vi "Read ADU Packet Slave.vi"(7 "Slave (F)":bool, 8 "error in (no error)":errorcluster, 10 "Transaction ID WR":u16, 11 "TCP in":refnum<class "TCP.lvclass">) -> (0 "error out":errorcluster, 1 "Modbus Data Unit":T2={"function"=1, "Data"=[]} {"function" items=["Read Discrete Inputs"=2, "Read Coils"=1, "Write Single Coil"=5, "Write Multiple Coils"=15, "Read Input Register"=4, "Read Holding Registers"=3, "Write Single Register"=6, "Write Multiple Registers"=16, "Read/Write Multiple Registers"=23, "Mask Write Register"=22, "Read FIFO Queue"=24, "Read File Record"=20, "Write File Record"=21, "Read Exception Status"=7, "Diagnostic"=8, "Get Com Event Counter"=11, "Get Com Event Log"=12, "Report Slave ID"=17, "Read Device Identification"=43]; "Data" format="%.0x"}, 2 "MBAP Header":T1, 3 "TCP out":refnum<class "TCP.lvclass">, 5 "PDU Valid?":bool)   [LabVIEW 2019]
doc: "This uses the protocol layer to read a modbus packet off of the bus, wrapped in the IP transmission data unit."
uses:
  <vilib>/ErrorRing/Error Ring.xnode
  <vilib>/Utility/error.llb/Error Cluster From Error Code.vi
  TCP/TCP.lvclass
  NI_modbus_upd.lvlib
  Ctl/MB Modbus Data Unit.ctl
  Modbus Functions/Function.ctl
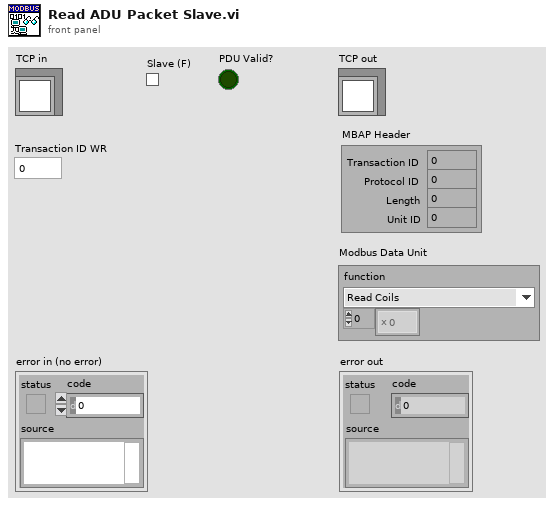
[diagram p1: front panel]
types:
  T1 = cluster{"Transaction ID":u16, "Protocol ID":u16, "Length":u16, "Unit ID":u8}
  T2 = typedef "NI_modbus_upd.lvlib/MB Modbus Data Unit.ctl" = cluster{"function":T3, "Data":u8[]}
  T3 = typedef "NI_modbus_upd.lvlib/Function.ctl" = u8
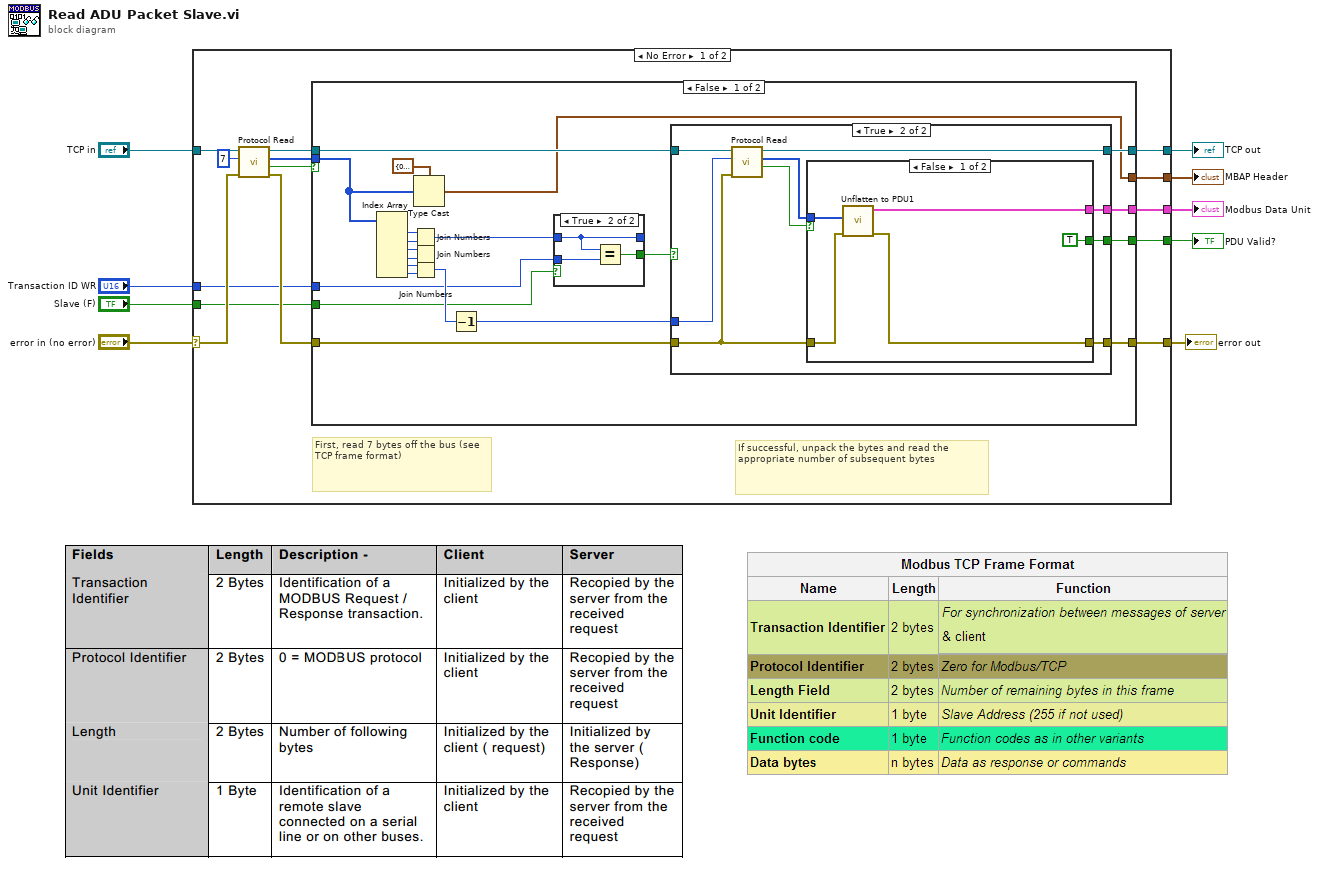
[diagram p0: block diagram]
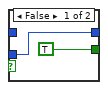
[diagram p2: hidden frame]
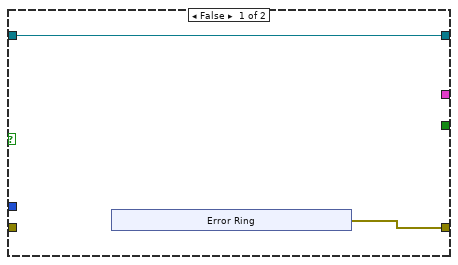
[diagram p3: hidden frame]
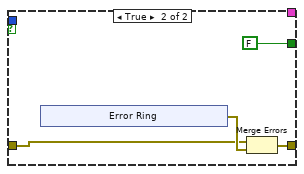
[diagram p4: hidden frame]
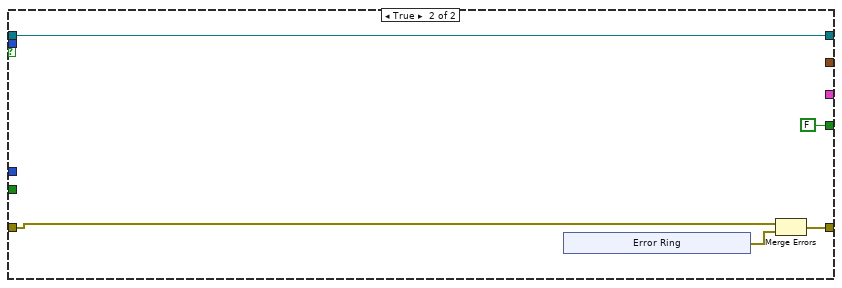
[diagram p5: hidden frame]
diagram:
  n1 = case shown="No Error" "error in (no error)" {
    selector: "error in (no error)" -> [w15 w88]
    tunnel: [w22 w88] -> w8
    tunnel: "TCP in" -> [w19 w87]
    tunnel: [w23 w87] -> w2
    tunnel: [w21 _] -> w3
    tunnel: [w20 _] -> w6
    tunnel: "Transaction ID WR" -> [w12 _]
    tunnel: "Slave (F)" -> [w11 _]
    tunnel: [w10 _] -> w1
    frame No Error {
      # "If successful, unpack the bytes and read the appropriate number of subsequent bytes"
      # "First, read 7 bytes off the bus (see TCP frame format)"
      n2 = call "Protocol Read.vi"("error in (no error)"=w15, "bytes to read"=7, "TCP in"=w19) -> ("error out"=w14:errorcluster, "timed out?"=w17:bool, "data"=w16:u8[], "TCP out"=w13:refnum<class "TCP.lvclass">)  [unwired: 5 in]
      n3 = case shown="False" w17 {
        tunnel: w16 -> [w25 _]
        tunnel: w13 -> [w28 w82]
        tunnel: [w27 w82] -> w23
        tunnel: w14 -> [w30 w79]
        tunnel: [w36 w80] -> w22
        tunnel: [w35 _] -> w21
        tunnel: [w34 FALSE] -> w20
        tunnel: w12 -> [w29 _]
        tunnel: w11 -> [w31 _]
        tunnel: [w24 _] -> w10
        frame False {
          n4 = Index Array(array=w25) -> (element #1=w43:u8, element #2=w44:u8, element #3=w42:u8, element #4=w41:u8, element #5=w39:u8, element #6=w40:u8)  [unwired: 6 in]
          n5 = Join Numbers(hi=w43, lo=w44) -> ((hi.lo)=w33:u16)
          n6 = Join Numbers(hi=w42, lo=w41) -> ()  [unwired: 1 out]
          n7 = Join Numbers(hi=w39, lo=w40) -> ((hi.lo)=w38:u16)
          n8 = Type Cast(type=T1 {"Transaction ID"=0, "Protocol ID"=0, "Length"=0, "Unit ID"=0} ("MBAP Header"), x=w25) -> (*(type *) &x=w24:T1)
          n9 = Decrement(x=w38) -> (x-1=w37:u16)
          n10 = case shown="True" w31 {
            tunnel: w33 -> [_ w47]
            tunnel: [TRUE w49] -> w32
            tunnel: w29 -> [w45 w48]
            tunnel: [w45 w47] -> _
            frame False {
            }
            frame True {
              n11 = Equal?(x=w47, y=w48) -> (x = y?=w49:bool)
            }
          }
          n12 = case shown="True" w32 {
            tunnel: w37 -> [_ w60]
            tunnel: [w51 w64] -> w36
            tunnel: [_ w63] -> w35
            tunnel: [_ w62] -> w34
            tunnel: w30 -> [_ w56]
            tunnel: w28 -> [w50 w61]
            tunnel: [w50 w57] -> w27
            frame False {
              n13 = xnode "Error Ring"() -> ("error out"=w51:errorcluster)
            }
            frame True {
              n14 = call "Protocol Read.vi"("error in (no error)"=w56, "bytes to read"=w60, "TCP in"=w61) -> ("timed out?"=w59:bool, "data"=w58:u8[], "TCP out"=w57:refnum<class "TCP.lvclass">)  [unwired: 5 in, 1 out]
              n15 = case shown="False" w59 {
                tunnel: [w65 w73] -> w64
                tunnel: [w68 _] -> w63
                tunnel: w58 -> [w67 _]
                tunnel: [TRUE FALSE] -> w62
                tunnel: w56 -> [w66 w70]
                frame False {
                  n16 = call "Unflatten to PDU1.vi"("error in (no error)"=w66, "Modbus data unit data"=w67) -> ("error out"=w65:errorcluster, "Modbus data unit out"=w68:T2)  [unwired: 8 in]
                }
                frame True {
                  n17 = xnode "Error Ring"() -> ("error out"=w72:errorcluster)
                  n18 = Merge Errors(w70, w72) -> (w73:errorcluster)
                }
              }
            }
          }
        }
        frame True {
          n19 = xnode "Error Ring"() -> ("error out"=w81:errorcluster)
          n20 = Merge Errors(w79, w81) -> (w80:errorcluster)
        }
      }
    }
    frame Error {
    }
  }
  "error out" <- w8
  "PDU Valid?" <- w6
  "MBAP Header" <- w1
  "Modbus Data Unit" <- w3
  "TCP out" <- w2
